vi "Update Moved Steps.vi"(8 "New Step Number":i32, 9 "Previous Step Number":i32, 11 "UI Data In":refnum<class "Settings UI.lvclass">) -> (3 "UI Data Out":refnum<class "Settings UI.lvclass">)   [LabVIEW 2020, in "Output Sequencer.lvlib" / "Settings UI.lvclass"]
uses:
  Settings UI.lvclass
  Settings UI.lvclass/Settings UI.ctl
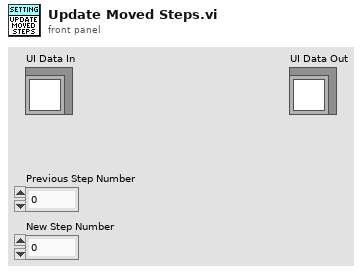
[diagram p1: front panel]
types:
  T1 = map{i32, cluster{"Step Number":i32, "Description":string}}
  T2 = typedef "Output Sequencer.lvlib/Settings UI.lvclass/Step Settings.ctl" = cluster{"Description":string, "Precondition":string, "Duration":dbl, "Mode":string, "Delay Between Values":dbl, "Analog Values":string[], "Digital Values":string[], "Postcondition":string, "On True":string, "On False":string}
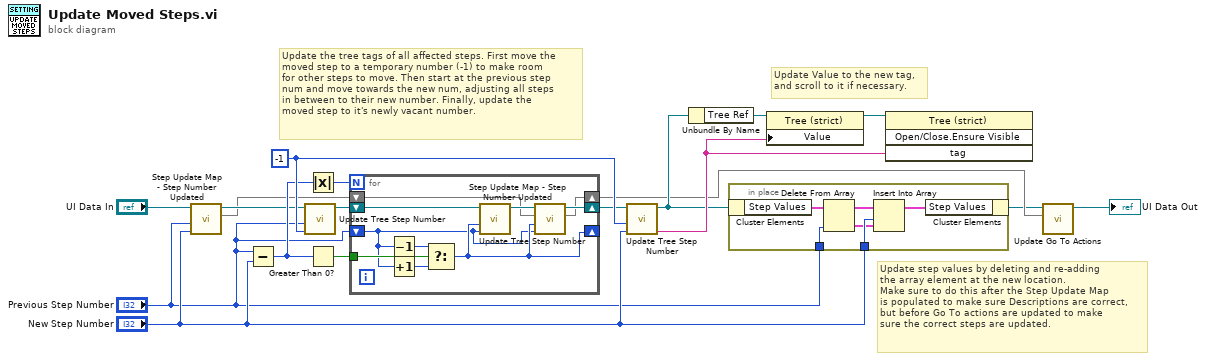
[diagram p0: block diagram]
diagram:
  w18 = -1 ("input 1")
  # "Update step values by deleting and re-adding\nthe array element at the new location.\nMake sure to do this after the Step Update Map\nis populated to make sure Descriptions are correct,\nbut before Go To actions are updated to make\nsure the correct steps are updated."
  # "Update the tree tags of all affected steps. First move the\nmoved step to a temporary number (-1) to make room\nfor other steps to move. Then start at the previous step\nnum and move towards the new num, adjusting all steps\nin between to their new number. Finally, update the\nmoved step to it's newly vacant number."
  # "Update Value to the new tag,\nand scroll to it if necessary."
  n1 = call "Step Update Map - Step Number Updated.vi"("New Step Number"="New Step Number", "Previous Step Number"="Previous Step Number", "Settings UI in"="UI Data In") -> ("Step Update Map out"=w3:T1, "Settings UI out"=w12:refnum<class "Settings UI.lvclass">)  [unwired: 7 in]
  n2 = Subtract(x="Previous Step Number", y="New Step Number") -> (x-y=w15:i32)
  n3 = call "Update Tree Step Number.vi"("New Step Number"=w18, "Old Step Number"="Previous Step Number", "UI Data In"=w12) -> ("UI Data Out"=w16:refnum<class "Settings UI.lvclass">)  [unwired: 6 in, 2 out]
  n4 = Absolute Value(x=w15) -> (abs(x)=w9:i32)
  n5 = Greater Than 0?(x=w15) -> (x > 0?=w8:bool)
  n6 = for {
    N: w9 -> [_]
    shift-right: [w23] -> w17
    shift-left: w16 -> [w28]
    shift-right: [w20] -> _
    shift-left: "Previous Step Number" -> [w19]
    tunnel: w8 -> [w27]
    shift-right: [w22] -> w2
    shift-left: w3 -> [w21]
    n7 = Decrement(x=w19) -> (x-1=w26:i32)
    n8 = Increment(x=w19) -> (x+1=w25:i32)
    n9 = Select(t=w26, s=w27, f=w25) -> (s? t:f=w20:i32)
    n10 = call "Update Tree Step Number.vi"("New Step Number"=w19, "Old Step Number"=w20, "UI Data In"=w28) -> ("UI Data Out"=w24:refnum<class "Settings UI.lvclass">)  [unwired: 6 in, 2 out]
    n11 = call "Step Update Map - Step Number Updated.vi"("New Step Number"=w19, "Previous Step Number"=w20, "Step Update Map in"=w21, "Settings UI in"=w24) -> ("Step Update Map out"=w22:T1, "Settings UI out"=w23:refnum<class "Settings UI.lvclass">)  [unwired: 6 in]
  }
  n12 = call "Update Tree Step Number.vi"("New Step Number"="New Step Number", "Old Step Number"=w18, "UI Data In"=w17) -> ("New Tag"=w13:string, "UI Data Out"=w4:refnum<class "Settings UI.lvclass">)  [unwired: 6 in, 1 out]
  n13 = Unbundle By Name(w4) -> ("Tree Ref"=w11:refnum<vi>)
  n14 = in-place {
    in-place-border: "New Step Number" -> [w34]
    in-place-border: "Previous Step Number" -> [w33]
    n15 = in-place-cluster #1(w4) -> ("Step Values"=w29:T2[])
    n16 = Delete From Array(array=w29, index=w33) -> (deleted portion=w32:T2, array with subset deleted=w31:T2[])  [unwired: 1 in]
    n17 = Insert Into Array(array=w31, index=w34, new element=w32) -> (w30:T2[])
    n18 = in-place-cluster #1("Step Values"=w30) -> (w1:refnum<class "Settings UI.lvclass">)
  }
  n19 = property class="Tree (strict)"(reference=w11, "Value"=w13) -> (reference out=w14:refnum<vi>)  [unwired: 1 in, 1 out]
  n20 = invoke class="Tree (strict)" method="Open/Close.Ensure Visible"(reference=w14, "tag"=w13) -> ()  [unwired: 2 in, 4 out]
  n21 = call "Update Go To Actions.vi"("Step Update Map in"=w2, "Settings UI in"=w1) -> ("Settings UI out"=→"UI Data Out":refnum<class "Settings UI.lvclass">)  [unwired: 9 in]
